vi "DataFile_Append.vi"(8 "iteration":i32, 10 "DataCluster":T1={"Core"={"Current VI Reference"=refnum, "Close Panel on Exit?"=FALSE, "Exit"=FALSE, "Initialized?"=FALSE}, "Connections"={"cDAQ"={"Task"="", "Connected"=FALSE, "Active"=FALSE, "ID"=""}, "Camera"={"Session"="", "Connected"=FALSE, "Active"=FALSE, "Placeholder"=refnum}, "PSU"={"Port"="", "Connected"=FALSE, "Active"=FALSE}, "Arduino"={"Port"="", "Connected"=FALSE, "Active"=FALSE}}, "Data Acquisition"={"Setup"={"Label"="", "Operator"="", "Notes"="", "TempGrad"=1.0, "TargetTemp"=1.0, "Sample Volume"=1.0}, "Camera"={"Image"=refnum, "Save Image"=refnum, "Image Frequency"=20, "Rectangle"={"Left"=0, "Top"=0, "Right"=0, "Bottom"=0, "Rotation"=0.0}, "Calibration"={"Top Left"={"X"=0.0, "Y"=0.0}, "Top Right"={"X"=0.0, "Y"=0.0}, "Bottom Left"={"X"=0.0, "Y"=0.0}, "Bottom Right"={"X"=0.0, "Y"=0.0}, "Fixpoint"={"X"=0.0, "Y"=0.0}, "Scan Area"=0.0, "Fixpoint Area"=0.0, "Well Pixels"=[], "Valid"=FALSE}, "FocusPos"=0, "Display Mapping"=10, "Camera Mode"=10}, "Thermistor"={"Sample Size"=1, "Calibration"={"B0.100"=[], "R25"=[], "c"=[], "State"=[], "V_S"=5.0, "R_S"=100.0}, "Timing Mode"=14713}, "Partition"={"Data"=[], "Cell Label"="", "Cell Color"=0, "Height"=10, "Width"=16, "Grid"=[]}, "Queue"={"Size"=1, "Queue"=refnum}, "Sample Rate"=1, "Active"=FALSE, "Ready"=FALSE, "Graph Mode"=0, "Gradient Buffer"=2}, "Control"={"Sample Rate"=1, "PID gains"={"proportional gain (Kc)"=1.0, "integral time (Ti, min)"=0.01, "derivative time (Td, min)"=0.0}}, "Manual Temp Control"={"TargetTemp"=1.0, "Mode"=0, "Active"=FALSE}} {"Manual Temp Control"."Mode" items=["Cool", "Heat"]; "Manual Temp Control"."TargetTemp" min=-40.0 max=40.0 step=0.5 format="%#_g °C"; "Control"."PID gains"."derivative time (Td, min)" format="%.3f"; "Control"."PID gains"."integral time (Ti, min)" format="%.3f"; "Control"."PID gains"."proportional gain (Kc)" format="%.3f"; "Control"."Sample Rate" min=1 max=20 step=1 format="%.0f Samples/sec"; "Data Acquisition"."Gradient Buffer" min=2 max=30 step=1; "Data Acquisition"."Graph Mode" items=["Thermistor Temperature", "Camera Temperature"]; "Data Acquisition"."Thermistor"."Timing Mode" items=["Automatic"=16097, "High Resolution"=10195, "High Speed"=14712, "Best 50 Hz Rejection"=14713, "Best 60 Hz Rejection"=14714, "Custom"=10137]; "Data Acquisition"."Thermistor"."Calibration"."R_S" min=0.1 max=1000.0 format="%#_g kOhm"; "Data Acquisition"."Thermistor"."Calibration"."V_S" min=5.0 max=48.0 format="%#_g V"; "Data Acquisition"."Thermistor"."Calibration"."R25" min=0.1 max=1000.0 format="%#_g kOhm"; "Data Acquisition"."Thermistor"."Calibration"."B0.100" min=100.0 max=10000.0 format="%#_g K"; "Data Acquisition"."Thermistor"."Sample Size" min=1 max=200; "Data Acquisition"."Sample Rate" min=20 max=240 format="%.0f samples/min"; "Data Acquisition"."Queue"."Size" min=1 max=200; "Data Acquisition"."Camera"."Camera Mode" items=["Temperature Linear", "Signal Linear"]; "Data Acquisition"."Camera"."Display Mapping" items=["Default"=10, "Most Significant Bits"=11, "Full Dynamic"=12, "Downshift"=13, "Given Range"=14, "90% Dynamic"=15, "Given Percent Range"=16]; "Data Acquisition"."Camera"."Calibration"."Fixpoint"."Y" format="%.2f"; "Data Acquisition"."Camera"."Calibration"."Fixpoint"."X" format="%.2f"; "Data Acquisition"."Camera"."Calibration"."Top Left"."Y" format="%.2f"; "Data Acquisition"."Camera"."Calibration"."Top Left"."X" format="%.2f"; "Data Acquisition"."Camera"."Calibration"."Top Right"."Y" format="%.2f"; "Data Acquisition"."Camera"."Calibration"."Top Right"."X" format="%.2f"; "Data Acquisition"."Camera"."Calibration"."Bottom Left"."Y" format="%.2f"; "Data Acquisition"."Camera"."Calibration"."Bottom Left"."X" format="%.2f"; "Data Acquisition"."Camera"."Calibration"."Bottom Right"."Y" format="%.2f"; "Data Acquisition"."Camera"."Calibration"."Bottom Right"."X" format="%.2f"; "Data Acquisition"."Camera"."Rectangle"."Rotation" min=-90.0 max=90.0 step=1.0 format="%.2f"; "Data Acquisition"."Camera"."Rectangle"."Left" scale=0.0..1024.0; "Data Acquisition"."Camera"."Rectangle"."Right" scale=0.0..1024.0; "Data Acquisition"."Camera"."Image Frequency" min=1 max=60 step=1; "Data Acquisition"."Setup"."Sample Volume" min=0.0 max=500.0 format="%#_g µL"; "Data Acquisition"."Setup"."TargetTemp" min=-40.0 max=40.0 step=0.5 format="%#_g °C"; "Data Acquisition"."Setup"."TempGrad" min=-100.0 max=100.0 step=0.1 format="%#_g °C/min"}) -> (0 "iteration out":i32)   [LabVIEW 2024]
uses:
  DataCluster.ctl
  <vilib>/userDefined/High Color/IMAQdx.ctl
  <vilib>/vision/Image Controls.llb/IMAQ Image.ctl
  <vilib>/Utility/file.llb/Write Delimited Spreadsheet (string).vi
panel:
  out "error out 2":errorcluster
  out "error out":errorcluster
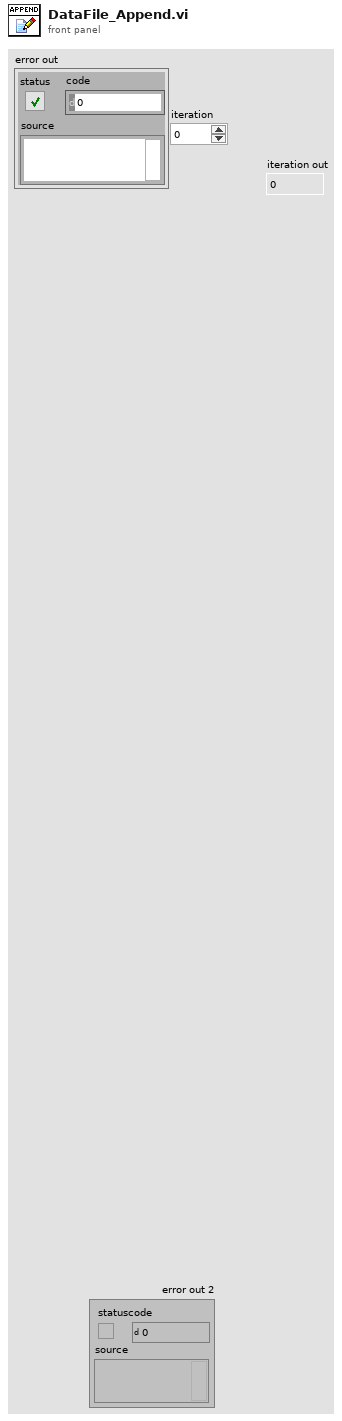
[diagram p1: front panel]
types:
  T1 = typedef "DataCluster.ctl" = cluster{"Core":cluster{"Current VI Reference":refnum<vi>, "Close Panel on Exit?":bool, "Exit":bool, "Initialized?":bool}, "Connections":cluster{"cDAQ":cluster{"Task":refnum<k21>, "Connected":bool, "Active":bool, "ID":string}, "Camera":cluster{"Session":T2, "Connected":bool, "Active":bool, "Placeholder":T3}, "PSU":cluster{"Port":refnum<visa-resource-name>, "Connected":bool, "Active":bool}, "Arduino":cluster{"Port":refnum<visa-resource-name>, "Connected":bool, "Active":bool}}, "Data Acquisition":cluster{"Setup":cluster{"Label":string, "Operator":string, "Notes":string, "TempGrad":dbl, "TargetTemp":dbl, "Sample Volume":dbl}, "Camera":cluster{"Image":T3, "Save Image":T3, "Image Frequency":i32, "Rectangle":T4, "Calibration":cluster{"Top Left":T5, "Top Right":T5, "Bottom Left":T5, "Bottom Right":T5, "Fixpoint":T5, "Scan Area":dbl, "Fixpoint Area":dbl, "Well Pixels":cluster{"X":i32, "Y":i32}[][], "Valid":bool}, "FocusPos":u32, "Display Mapping":u32, "Camera Mode":u32}, "Thermistor":cluster{"Sample Size":i32, "Calibration":cluster{"B0.100":dbl[], "R25":dbl[], "c":dbl[][], "State":bool[], "V_S":dbl, "R_S":dbl}, "Timing Mode":i32}, "Partition":cluster{"Data":string[][], "Cell Label":string, "Cell Color":u32, "Height":i32, "Width":i32, "Grid":string[][]}, "Queue":cluster{"Size":i32, "Queue":refnum<queue>}, "Sample Rate":i32, "Active":bool, "Ready":bool, "Graph Mode":u16, "Gradient Buffer":i32}, "Control":cluster{"Sample Rate":i32, "PID gains":cluster{"proportional gain (Kc)":dbl, "integral time (Ti, min)":dbl, "derivative time (Td, min)":dbl}}, "Manual Temp Control":cluster{"TargetTemp":dbl, "Mode":u16, "Active":bool}}
  T2 = typedef "IMAQdx.ctl" = refnum<k21>
  T3 = typedef "IMAQ Image.ctl" = refnum<image>
  T4 = typedef "IMAQ Rectangle" = cluster{"Left":i32, "Top":i32, "Right":i32, "Bottom":i32, "Rotation":dbl}
  T5 = typedef "IMAQ Point" = cluster{"X":sgl, "Y":sgl}
  T6 = cluster{"Mean Temperature":dbl, "Temp Gradient":dbl, "Temperature Readings":dbl[], "Voltage Readings":dbl[], "Temp Std":dbl[], "Image Pixels (U32)":u16[][], string}
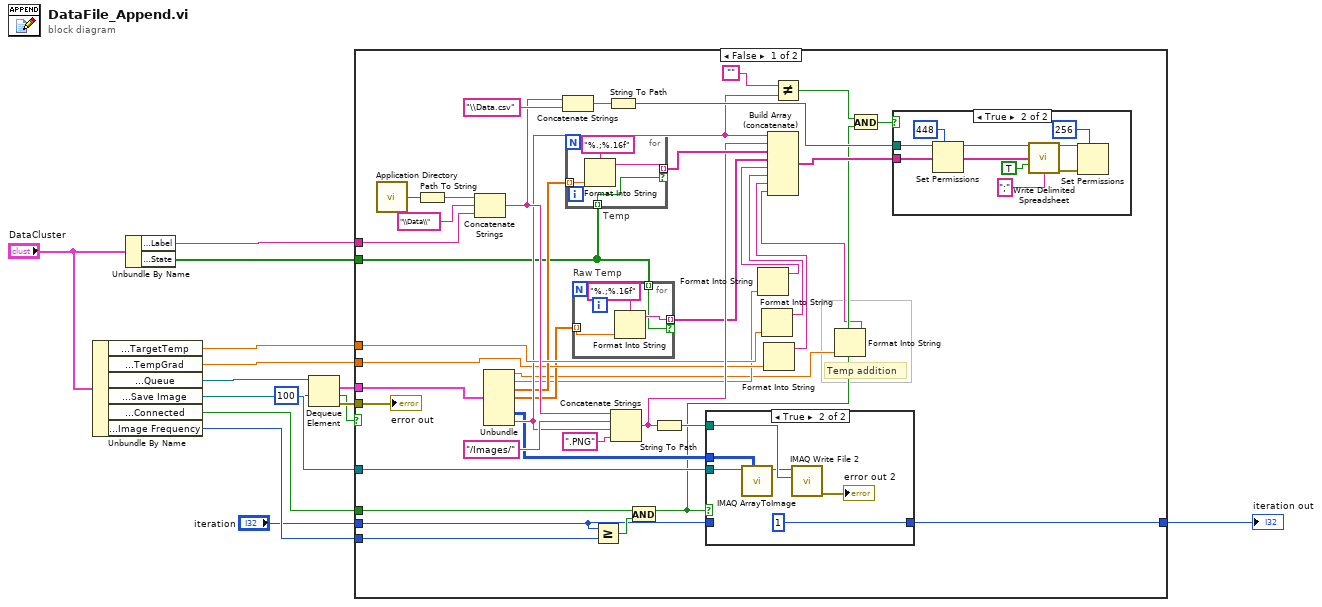
[diagram p0: block diagram]
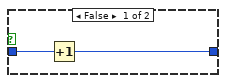
[diagram p2: hidden frame]
diagram:
  n1 = Unbundle By Name("DataCluster") -> ("Data Acquisition.Setup.TargetTemp"=w5:dbl, "Data Acquisition.Setup.TempGrad"=w4:dbl, "Data Acquisition.Queue.Queue"=w13:refnum<queue>, "Data Acquisition.Camera.Save Image"=w11:T3, "Connections.Camera.Connected"=w10:bool, "Data Acquisition.Camera.Image Frequency"=w8:i32)
  n2 = Unbundle By Name("DataCluster") -> ("Data Acquisition.Setup.Label"=w15:string, "Data Acquisition.Thermistor.Calibration.State"=w3:bool[])
  n3 = Dequeue Element(queue=w13, timeout in ms (-1)=100) -> (element=w12:T6, timed out?=w1:bool, error out=w9:errorcluster)  [unwired: 1 in, 1 out]
  n4 = case shown="False" w1 {
    tunnel: w15 -> [w52 _]
    tunnel: w12 -> [w49 _]
    tunnel: w11 -> [w47 _]
    tunnel: w10 -> [w40 _]
    tunnel: w9 -> [w39 _]
    tunnel: w8 -> [w34 _]
    tunnel: "iteration" -> [w33 w81]
    tunnel: [w32 w81] -> w6
    tunnel: w5 -> [w29 _]
    tunnel: w4 -> [w25 _]
    tunnel: w3 -> [w23 _]
    frame False {
      # "Temp addition"
      n5 = call <vilib>:"Application Directory.vi"() -> ("Application Directory"=w55:path)
      n6 = Path To String(path=w55) -> (string=w54:string)
      n7 = Concatenate Strings(w54, "\\Data\\", w52) -> (w36:string)
      n8 = Unbundle(w49) -> ("Mean Temperature"=w17:dbl, "Temp Gradient"=w19:dbl, "Temperature Readings"=w26:dbl[], "Voltage Readings"=w20:dbl[], "Image Pixels (U32)"=w27:u16[][], w28:string)  [unwired: 1 out]
      n9 = Concatenate Strings(w36, "\\Data.csv") -> (w46:string)
      n10 = for "Temp" {
        tunnel: w26 -> [w80] mode=indexing
        tunnel: [w79] -> w50 mode=indexing if=w78
        tunnel: w23 -> [w78] mode=indexing
        n11 = Format Into String(format string="%.;%.16f", w80) -> (resulting string=w79:string)  [unwired: 2 in, 1 out]
      }
      n12 = for "Raw Temp" {
        tunnel: [w59] -> w24 mode=indexing if=w58
        tunnel: w23 -> [w58] mode=indexing
        tunnel: w20 -> [w57] mode=indexing
        n13 = Format Into String(format string="%.;%.16f", w57) -> (resulting string=w59:string)  [unwired: 2 in, 1 out]
      }
      n14 = Greater Or Equal?(x=w33, y=w34) -> (x >= y?=w35:bool)
      n15 = String To Path(string=w46) -> (path=w51:path)
      n16 = Concatenate Strings(w36, "/Images/" ("string"), w28, ".PNG" ("string")) -> (w41:string)
      n17 = And(x=w40, y=w35) -> (x .and. y?=w21:bool)
      n18 = String To Path(string=w41) -> (path=w43:path)
      n19 = case shown="True" w21 {
        tunnel: w27 -> [_ w62]
        tunnel: w47 -> [_ w64]
        tunnel: w43 -> [_ w67]
        tunnel: w33 -> [w61 _]
        tunnel: [w60 1] -> w32
        frame False {
          n20 = Increment(x=w61) -> (x+1=w60:i32)
        }
        frame True {
          n21 = call "IMAQ ArrayToImage"("Image Pixels (U16)"=w62, "Image"=w64) -> ("Image Out"=w63:T3)  [unwired: 8 in, 1 out]
          n22 = call-poly "IMAQ Write File 2"("File Path"=w67, "Image"=w63) -> ("error out"=→"error out 2":errorcluster)  [unwired: 8 in, 1 out]
        }
      }
      n23 = Format Into String(w19) -> (resulting string=w31:string)  [unwired: 3 in, 1 out]
      n24 = Format Into String(w29) -> (resulting string=w30:string)  [unwired: 3 in, 1 out]
      n25 = Format Into String(w25) -> (resulting string=w18:string)  [unwired: 3 in, 1 out]
      n26 = Not Equal?(x="", y=w28) -> (x != y?=w37:bool)
      n27 = Format Into String(w17) -> (resulting string=w16:string)  [unwired: 3 in, 1 out]
      n28 = Build Array (concatenate)(w28, w41, w50, w24, w31, w30, w18, w16) -> (w42:string[])
      n29 = And(x=w37, y=w21) -> (x .and. y?=w22:bool)
      n30 = case shown="True" w22 {
        tunnel: w51 -> [_ w73]
        tunnel: w42 -> [_ w74]
        frame False {
        }
        frame True {
          n31 = Set Permissions(7:i16 448 ("permissions"), 11:w73) -> (3:w72:path)  [unwired: 3 in, 1 out]
          n32 = call-poly <vilib>:"Write Delimited Spreadsheet.vi"("file path (dialog if empty)"=w72, "1D data"=w74, "append to file? (new file:F)"=TRUE, "delimiter (\\t)"=";" ("delimiter (\\t)")) -> ("new file path (Not A Path if cancelled)"=w71:path, "error out"=w70:errorcluster)  [unwired: 10 in]
          n33 = Set Permissions(7:i16 256 ("permissions"), 8:w70, 11:w71) -> ()  [unwired: 2 in, 2 out]
        }
      }
      "error out" <- w39
    }
    frame True {
    }
  }
  "iteration out" <- w6
